vi "EMC_ABS_Move.vi"(8 "error in (no error)":errorcluster, 10 "Motion Parameters":T1={"position"=1000.0, "velocity"=1000.0, "acceleration"=10000.0, "deceleration"=10000.0, "accel. jerk"=10000.0, "decel. jerk"=10000.0}, 11 "axis":refnum<k21>) -> (0 "error out":errorcluster)   [LabVIEW 2015]
uses:
  EMC_Typedef_Motor_Parameters.ctl
  <vilib>/Motion/PropertyNodes/nimc.createStraightLineMoveInstance.axis.vi
  <vilib>/Motion/PropertyNodes/nimc.destroyInterfaceInstance.vi
  <resource>/objmgr/nimotion.rc
panel:
  out "Numeric":i32
  in  "table":refnum<k21>
  in  "coordinate":refnum<k21>
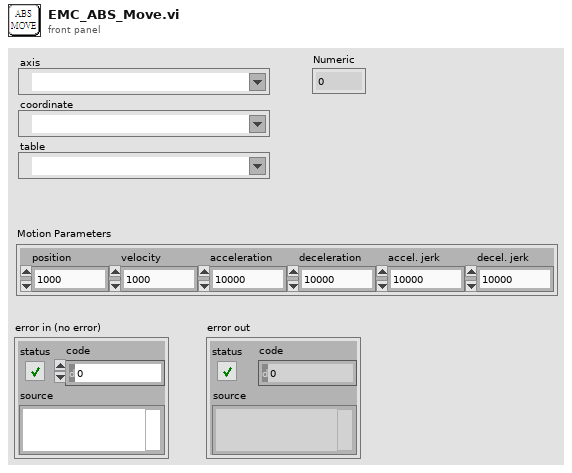
[diagram p1: front panel]
types:
  T1 = typedef "EMC_Typedef_Motor_Parameters.ctl" = cluster{"position":dbl, "velocity":dbl, "acceleration":dbl, "deceleration":dbl, "accel. jerk":dbl, "decel. jerk":dbl}
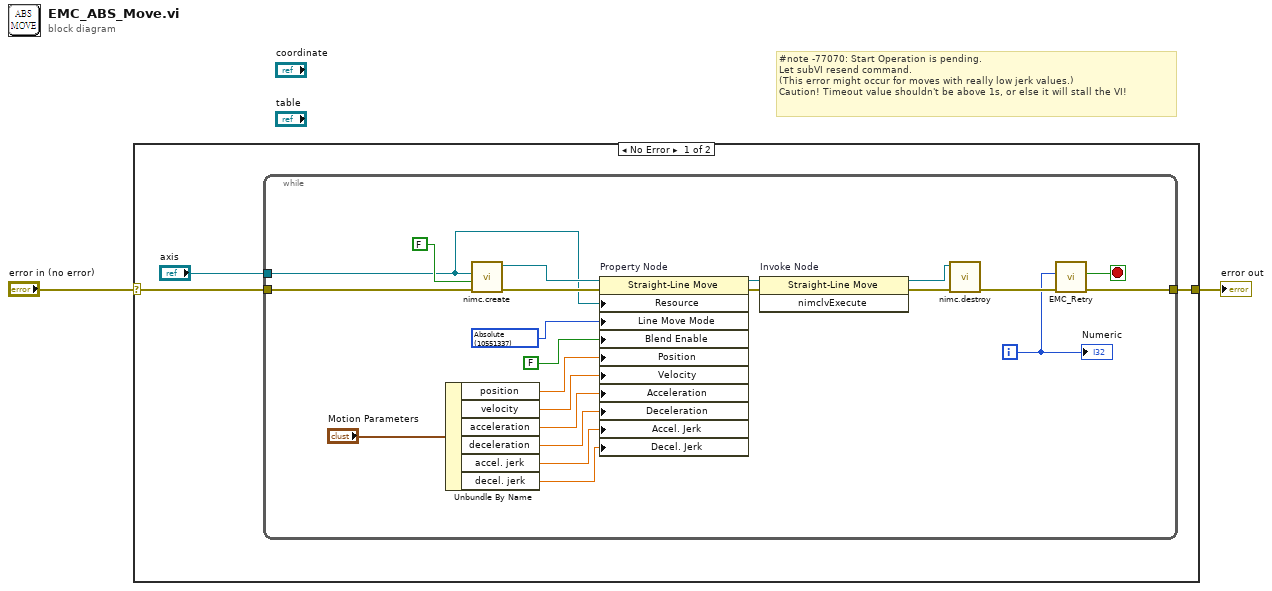
[diagram p0: block diagram]
diagram:
  # "#note -77070: Start Operation is pending.\nLet subVI resend command.\n(This error might occur for moves with really low jerk values.)\nCaution! Timeout value shouldn't be above 1s, or else it will stall the VI!"
  n1 = case shown="No Error" "error in (no error)" {
    selector: "error in (no error)" -> [w4 w28]
    tunnel: [w5 w28] -> w2
    frame No Error {
      n2 = while {
        tunnel: [w6] -> w5
        tunnel: w4 -> [w11]
        tunnel: "axis" -> [w10]
        i -> [w8]
        stop <- w7 stop-if-true
        w12 = 10551337 items=["Relative"=10551344, "Absolute"=10551337, "Relative To Capture"=10551345, "Velocity"=10551346, "Polyline"=11600101] ("line move mode")
        n3 = Unbundle By Name("Motion Parameters") -> ("position"=w18:dbl, "velocity"=w17:dbl, "acceleration"=w16:dbl, "deceleration"=w15:dbl, "accel. jerk"=w14:dbl, "decel. jerk"=w13:dbl)
        n4 = call-poly <vilib>:"nimc.create.vi"("error in"=w11, "async?"=FALSE ("execute asynchronously?"), "axis"=w10) -> ("error out"=w24:errorcluster, "line"=w20:refnum<k20>)  [unwired: 6 in, 1 out]
        n5 = property on="Property Node" class="Straight-Line Move"(reference=w20, error in=w24, "Resource"=w10, "Line Move Mode"=w12, "Blend Enable"=FALSE ("blend enable"), "Position"=w18, "Velocity"=w17, "Acceleration"=w16, "Deceleration"=w15, "Accel. Jerk"=w14, "Decel. Jerk"=w13) -> (reference out=w27:refnum<k20>, error out=w26:errorcluster)
        n6 = invoke on="Invoke Node" class="Straight-Line Move" method="nimclvExecute"(reference=w27, error in=w26) -> (reference out=w23:refnum<k20>, error out=w22:errorcluster)  [unwired: 1 in, 1 out]
        n7 = call-poly <vilib>:"nimc.destroy.vi"("error in"=w22, "motion handle"=w23) -> ("error out"=w9:errorcluster)  [unwired: 9 in]
        n8 = call "EMC_Retry.vi"("error in (no error)"=w9, "Count in"=w8) -> ("error out"=w6:errorcluster, "Exit"=w7:bool)  [unwired: 8 in]
        "Numeric" <- w8
      }
    }
    frame Error {
    }
  }
  "error out" <- w2
